vi "Covert Header to Package Layer.vi"(11 "Ethernet Header Cluster":T2 {"Ethertype" format="%.0x"; "VLAN Tag"."VID" format="%.0x"; "VLAN Tag"."TPID" format="%.0x"; "source MAC address"."?" format="%02x"; "source MAC address"."?" format="%02x"; "source MAC address"."?" format="%02x"; "source MAC address"."?" format="%02x"; "source MAC address"."?" format="%02x"; "source MAC address"."?" format="%02x"; "destination MAC address"."?" format="%02x"; "destination MAC address"."?" format="%02x"; "destination MAC address"."?" format="%02x"; "destination MAC address"."?" format="%02x"; "destination MAC address"."?" format="%02x"; "destination MAC address"."?" format="%02x"}) -> (3 "Protocol Layer":T1)   [LabVIEW 2025, in "Automotive Ethernet Bus Monitor UI.lvlib"]
doc: "Generates a Protocol Layer Cluster element from a Ethernet Header Cluster element."
uses:
  Automotive Ethernet Bus Monitor UI.lvlib
  Ethernet Header Cluster.ctl
  Protocol Layer.ctl
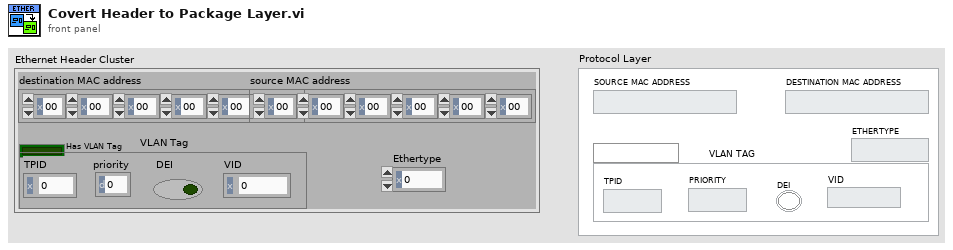
[diagram p1: front panel]
types:
  T1 = typedef "Automotive Ethernet Bus Monitor UI.lvlib/Protocol Layer.ctl" = cluster{"Has VLAN":bool, "VLAN TAG":cluster{"TPID":u16, "PRIORITY":u8, "DEI":bool, "VID":u16}, "SOURCE MAC ADDRESS":string, "DESTINATION MAC ADDRESS":string, "ETHERTYPE":u16}
  T2 = typedef "Automotive Ethernet Bus Monitor UI.lvlib/Ethernet Header Cluster.ctl" = cluster{"destination MAC address":cluster{u8, u8, u8, u8, u8, u8}, "source MAC address":cluster{u8, u8, u8, u8, u8, u8}, "Has VLAN Tag":bool, "VLAN Tag":cluster{"TPID":u16, "priority":u8, "DEI":bool, "VID":u16}, "Ethertype":u16}
  T3 = cluster{"TPID":u16, "priority":u8, "DEI":bool, "VID":u16}
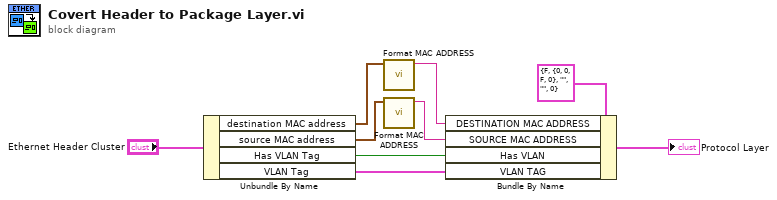
[diagram p0: block diagram]
diagram:
  n1 = Unbundle By Name("Ethernet Header Cluster") -> ("destination MAC address"=w7:cluster{u8, u8, u8, u8, u8, u8}, "source MAC address"=w9:cluster{u8, u8, u8, u8, u8, u8}, "Has VLAN Tag"=w3:bool, "VLAN Tag"=w4:T3)
  n2 = call "Format MAC ADDRESS.vi"("source MAC address"=w7) -> ("spreadsheet string"=w6:string)  [unwired: 10 in]
  n3 = call "Format MAC ADDRESS.vi"("source MAC address"=w9) -> ("spreadsheet string"=w8:string)  [unwired: 10 in]
  n4 = Bundle By Name(cluster=T1 {"Has VLAN"=FALSE, "VLAN TAG"={"TPID"=0, "PRIORITY"=0, "DEI"=FALSE, "VID"=0}, "SOURCE MAC ADDRESS"="", "DESTINATION MAC ADDRESS"="", "ETHERTYPE"=0} ("Protocol Layer"), "DESTINATION MAC ADDRESS"=w6, "SOURCE MAC ADDRESS"=w8, "Has VLAN"=w3, "VLAN TAG"=w4) -> (→"Protocol Layer":T1)
